vi "test_Create Global MetaData Channel_single channel format.vi"(8 "error in (no error)":errorcluster, 11 "TestCase in":refnum<class "Instrument Addon Scripting API Channels Unit Tests.lvclass">) -> (0 "error out":errorcluster, 3 "TestCase out":refnum<class "Instrument Addon Scripting API Channels Unit Tests.lvclass">)   [LabVIEW 2018, in "Instrument Addon Scripting API Channels Unit Tests.lvclass"]
uses:
  Instrument Addon Scripting API Channels Unit Tests.lvclass
  Addon/Addon Shared/Types/FG Control.ctl
  APIs/Scripting API/TypeDefs/Single Channel Format Settings.ctl
  Instrument Addon Scripting API Channels Unit Tests.lvclass/Instrument Addon Scripting API Channels Unit Tests.ctl
  Addon/Addon Shared/SubVIs/Constants.vi
  APIs/Scripting API/Channels/Create Global MetaData Channel - Single Channel - Format.vi
  <vilib>/NI Veristand/Custom Device Tools/Custom Device Utility Library/NI VeriStand - Search for Item by GUID.vi
  <vilib>/NI Veristand/Custom Device Tools/Custom Device Utility Library/NI VeriStand - Search for Item by Name.vi
  <vilib>/NI Veristand/Custom Device API/NI VeriStand - Get Item Property.vi
  <vilib>/NI Veristand/Custom Device API/Get Item Property (U32).vi
  <vilib>/NI Veristand/Custom Device API/Get Item Property (String Array).vi
  <vilib>/NI Veristand/Custom Device API/Get Item Property (String).vi
  <vilib>/NI Veristand/Custom Device API/NI VeriStand - Set Item Property.vi
  <vilib>/NI Veristand/Custom Device API/Set Item Property (U32).vi
  <vilib>/NI Veristand/Custom Device API/Set Item Property (String Array).vi
  <vilib>/NI Veristand/Custom Device API/NI VeriStand - Get Item Children.vi
  Addon/Addon Shared/SubVIs/Set Channel Value Table.vi
  <vilib>/NI Veristand/Custom Device API/Set Item Property (String).vi
  <vilib>/addons/_JKI Toolkits/VI Tester/TestCase.llb/TestCase.lvclass
  Instrument Addon Scripting API Test Assets/Instrument Addon Scripting API Test Assets.lvclass
  <vilib>/NI Veristand/Custom Device Tools/Custom Device Utility Library/Custom Device Utility Library.lvlib
  Addon/Addon Shared/Instrument Addon Shared.lvlib
  <vilib>/NI Veristand/Custom Device API/Custom Device API.lvlib
  APIs/Scripting API/Instrument Addon Scripting API.lvlib
  C:/Program Files (x86)/National Instruments/LabVIEW 2018/vi.lib/addons/_JKI Toolkits/VI Tester/TestCase.llb/TestCase.lvclass
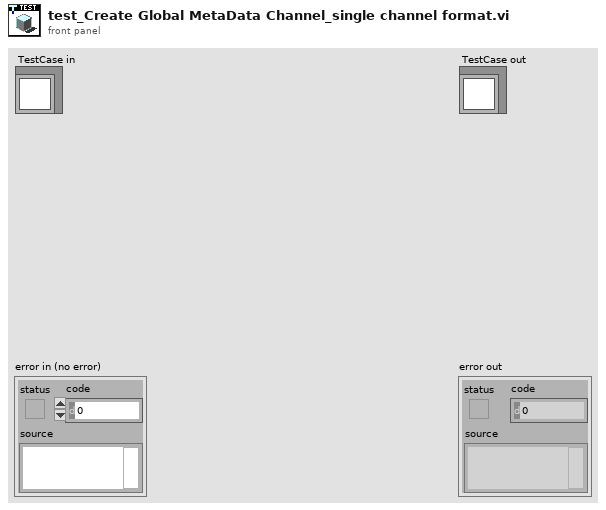
[diagram p1: front panel]
types:
  T1 = typedef "Instrument Addon Shared.lvlib/FG Control.ctl" = enum16{"Get", "Set"}
  T2 = typedef "Instrument Addon Scripting API.lvlib/Single Channel Format Settings.ctl" = cluster{"Format String":string, "Default Value":dbl, "Units":string}
  T3 = typedef "Custom Device API.lvlib/Custom Device Item Ref.ctl" = u64
  T4 = typedef "Instrument Addon Shared.lvlib/MetaData Parameters.ctl" = cluster{"Data Type":T5, "Channel Type":T6, "List":string[], "Format String":string, "Type":T7, "Delimiter":string, "Endian":T8}
  T5 = typedef "Instrument Addon Shared.lvlib/Protocol Data Type.ctl" = enum16{"Single Channel", "Array"}
  T6 = typedef "Instrument Addon Shared.lvlib/Metadata Channel Type.ctl" = enum16{"Enumerated List", "Format", "Type Cast"}
  T7 = typedef "Instrument Addon Shared.lvlib/Type Cast Type.ctl" = enum16{"DBL", "SGL", "U64", "U32", "U16", "U8", "I64", "I32", "I16", "I8"}
  T8 = typedef "Instrument Addon Shared.lvlib/Endian.ctl" = enum16{"Native", "Little", "Big"}
  T9 = typedef "Custom Device API.lvlib/Custom Device Channel.ctl" = cluster{"Type":T10, "Units":string, "Default Value":dbl, "Faultable":bool, "Scalable":bool}
  T10 = typedef "Custom Device API.lvlib/Custom Device Channel Type.ctl" = enum16{"Input", "Output"}
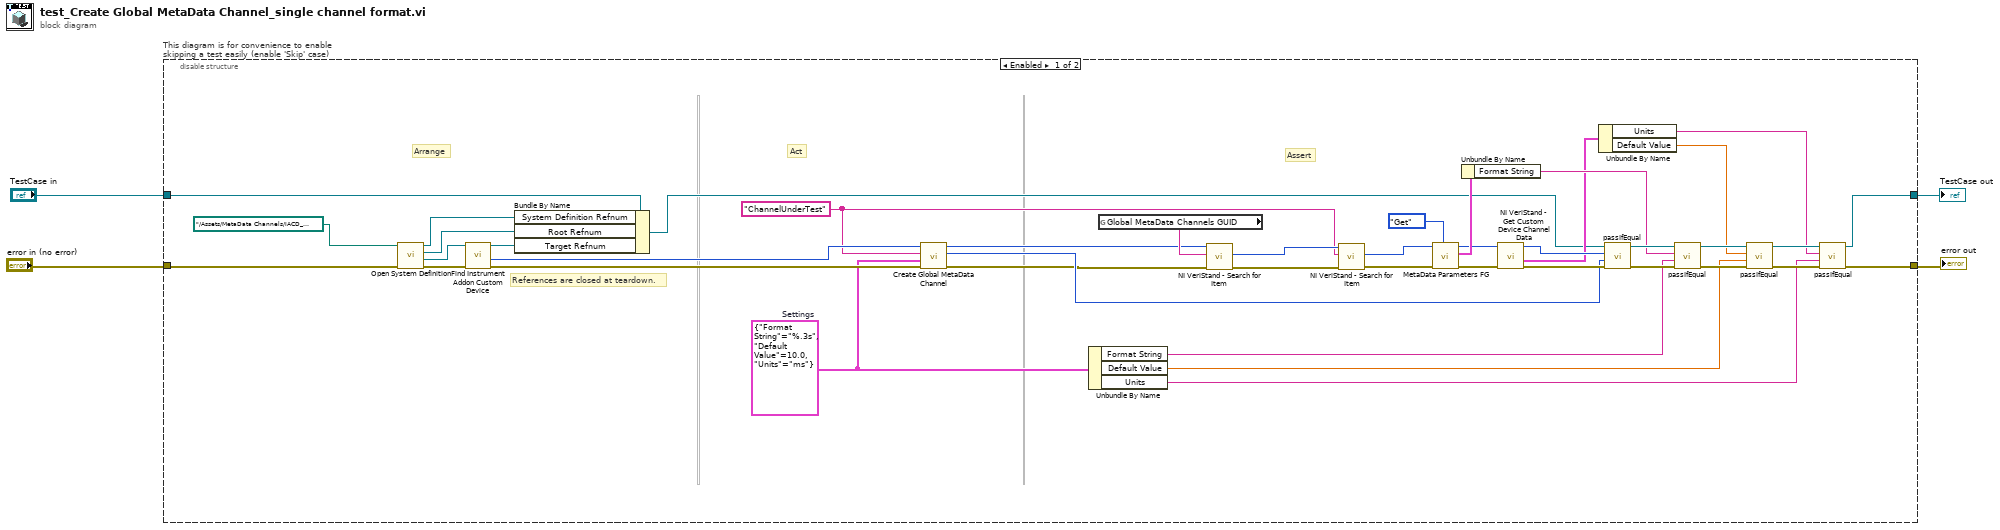
[diagram p0: block diagram]
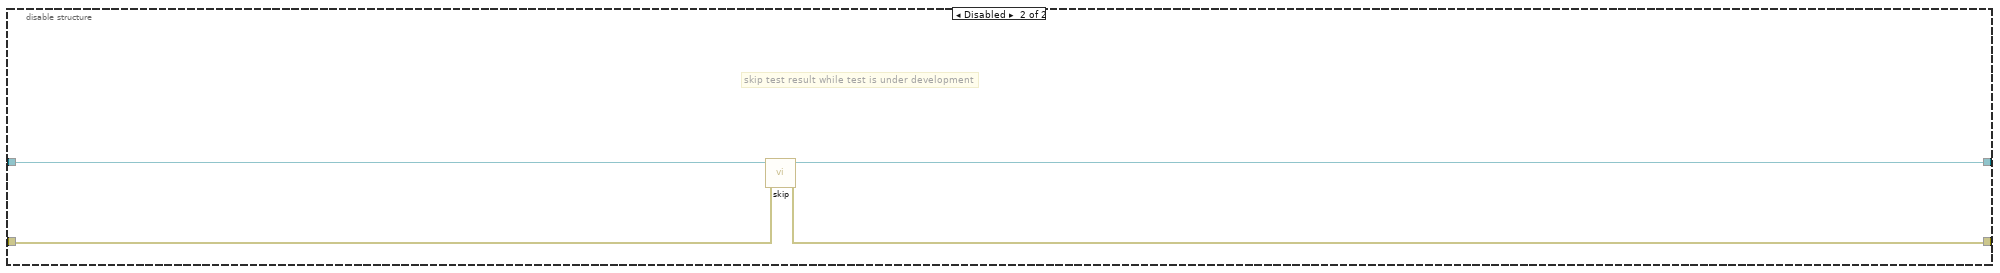
[diagram p2: hidden frame]
diagram:
  n1 = disable-structure "This diagram is for convenience to enable skipping a test easily (enable 'Skip' case)" shown="Enabled" {
    disable-tunnel: "TestCase in" -> [w13 w50]
    disable-tunnel: [w20 w48] -> w1
    disable-tunnel: [w19 w49] -> w3
    disable-tunnel: "error in (no error)" -> [w46 w47]
    frame Enabled {
      w6 = T2 {"Format String"="%.3s", "Default Value"=10.0, "Units"="ms"}  # Settings
      w11 = "ChannelUnderTest" ("Name")
      # "References are closed at teardown."
      # "Assert"
      # "Act"
      # "Arrange"
      n2 = call "Open System Definition.vi"("error in (no error)"=w46, "System Definition File"=path "../Assets/MetaData Channels/IACD_channels.nivssdf") -> ("error out"=w44:errorcluster, "Target Refnum"=w45:refnum<k24>, "Root Refnum"=w16:refnum<k24>, "System Definition Refnum"=w15:refnum<k24>)  [unwired: 6 in]
      n3 = call "Find Instrument Addon Custom Device.vi"("error in"=w44, "target in"=w45) -> ("error out"=w10:errorcluster, "NodeID"=w12:u64, "target out"=w17:refnum<k24>)  [unwired: 7 in]
      n4 = Bundle By Name(cluster=w13, "System Definition Refnum"=w15, "Root Refnum"=w16, "Target Refnum"=w17) -> (w14:refnum<class "Instrument Addon Scripting API Channels Unit Tests.lvclass">)
      n5 = call-poly "Create Global MetaData Channel.vi"("Error In"=w10, "Settings"=w6, "Name"=w11, "Instrument Addon Refnum In"=w12) -> ("Error Out"=w7:errorcluster, "Channel Refnum"=w8:T3, "Instrument Addon Refnum Out"=w9:T3)  [unwired: 5 in]
      n6 = Unbundle By Name(w6) -> ("Format String"=w29:string, "Default Value"=w25:dbl, "Units"=w24:string)
      n7 = global read "Constants.vi" "Global MetaData Channels GUID"() -> (w43:string)
      n8 = call-poly <vilib>:"NI VeriStand - Search for Item.vi"("error in"=w7, "Item GUID"=w43, "Section Ref in"=w9) -> ("error out"=w41:errorcluster, "Item Ref"=w42:T3)  [unwired: 5 in, 2 out]
      n9 = call-poly <vilib>:"NI VeriStand - Search for Item.vi"("error in"=w41, "Item Name"=w11, "Section Ref in"=w42) -> ("error out"=w40:errorcluster, "Item Ref"=w39:T3)  [unwired: 5 in, 2 out]
      n10 = call "MetaData Parameters FG.vi"("Action"=FG_Control."Get", "error in (no error)"=w40, "Item Ref in"=w39) -> ("error out"=w27:errorcluster, "MetaData Parameters"=w37:T4, "Item Ref out"=w28:T3)  [unwired: 6 in]
      n11 = Unbundle By Name(w37) -> ("Format String"=w30:string)
      n12 = call <vilib>:"NI VeriStand - Get Custom Device Channel Data.vi"("error in (no error)"=w27, "Channel Ref in"=w28) -> ("error out"=w18:errorcluster, "Channel"=w23:T9, "Channel Ref out"=w26:T3)  [unwired: 4 in, 3 out]
      n13 = Unbundle By Name(w23) -> ("Units"=w21:string, "Default Value"=w22:dbl)
      n14 = call-dynamic "passIfEqual.vi"("error in (no error)"=w18, "y"=w8, "x"=w26, "TestCase in"=w14) -> ("error out"=w36:errorcluster, "TestCase out"=w35:refnum<class "Instrument Addon Scripting API Channels Unit Tests.lvclass">)  [unwired: 6 in]
      n15 = call-dynamic "passIfEqual.vi"("error in (no error)"=w36, "y"=w29, "x"=w30, "TestCase in"=w35) -> ("error out"=w34:errorcluster, "TestCase out"=w33:refnum<class "Instrument Addon Scripting API Channels Unit Tests.lvclass">)  [unwired: 6 in]
      n16 = call-dynamic "passIfEqual.vi"("error in (no error)"=w34, "y"=w25, "x"=w22, "TestCase in"=w33) -> ("error out"=w32:errorcluster, "TestCase out"=w31:refnum<class "Instrument Addon Scripting API Channels Unit Tests.lvclass">)  [unwired: 6 in]
      n17 = call-dynamic "passIfEqual.vi"("error in (no error)"=w32, "y"=w24, "x"=w21, "TestCase in"=w31) -> ("error out"=w19:errorcluster, "TestCase out"=w20:refnum<class "Instrument Addon Scripting API Channels Unit Tests.lvclass">)  [unwired: 6 in]
    }
    frame Disabled {
      # "skip test result while test is under development"
      n18 = call <vilib>:"skip.vi"("error in (no error)"=w47, "TestCase in"=w50) -> ("error out"=w49:errorcluster, "TestCase out"=w48:refnum<class "Instrument Addon Scripting API Channels Unit Tests.lvclass">)  [unwired: 8 in]
    }
  }
  "error out" <- w3
  "TestCase out" <- w1
